vi "Resample.vi"(10 "Divide by":i32=20, 11 "Waveform":waveform(dbl)) -> (3 "output waveform":waveform(dbl))   [LabVIEW 2010]
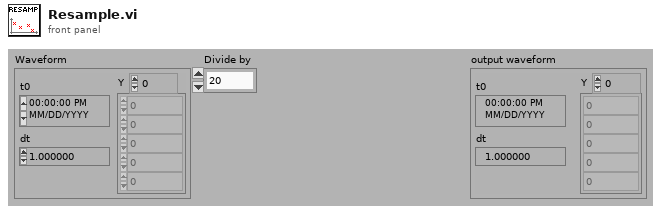
[diagram p1: front panel]
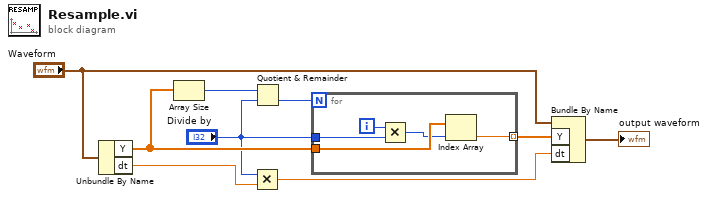
[diagram p0: block diagram]
diagram:
  n1 = Unbundle By Name("Waveform") -> ("Y"=w5:dbl[], "dt"=w7:dbl)
  n2 = Array Size(array=w5) -> (size(s)=w3:i32)
  n3 = Multiply(x="Divide by", y=w7) -> (x*y=w8:dbl)
  n4 = Quotient & Remainder(x=w3, y="Divide by") -> (floor(x/y)=w2:i32)  [unwired: 1 out]
  n5 = for {
    N: w2 -> [_]
    tunnel: w5 -> [w13]
    tunnel: [w11] -> w1 mode=indexing
    tunnel: "Divide by" -> [w10]
    i -> [w14]
    n6 = Multiply(x=w14, y=w10) -> (x*y=w12:i32)
    n7 = Index Array(array=w13, index=w12) -> (element=w11:dbl)
  }
  n8 = Bundle By Name(cluster="Waveform", "Y"=w1, "dt"=w8) -> (→"output waveform":waveform(dbl))
